vi "DMM.vi"(6 "Setting":T1={"Resolution (Digits)"=5.5, "Current Source (Amps)"=0.001, "Range"=2.0, "Measurement Type"=enum."DC Volts"} {"Resolution (Digits)" items=["3 1/2"=3.5, "4 1/2"=4.5, "5 1/2"=5.5, "6 1/2"=6.5, "7 1/2"=7.5]; "Current Source (Amps)" items=["1uA"=1e-06, "10uA"=1e-05, "100uA"=0.0001, "1mA"=0.001]}, 8 "error in":errorcluster, 9 "DMM Ref":string="NI_DMM_4072", 10 "DMM ClassName":string="NI DMM4072.lvclass", 11 "Base Path":path=path "C:/GitHub/OOP_OPC UA/Sequence/CodeModules/HAL/Concrete") -> (0 "error out":errorcluster={"status"=TRUE, "code"=-1073807346, "source"="VISA Open in APS-7000 Series.lvlib:Initialize.vi->Concrete.lvlib:APS7050.lvclass:Initialise.vi->Check objects.vi"}, 3 "Measurements":dbl)   [LabVIEW 2021]
uses:
  HAL/Harware Abstraction/MultiIO/DMM.lvclass
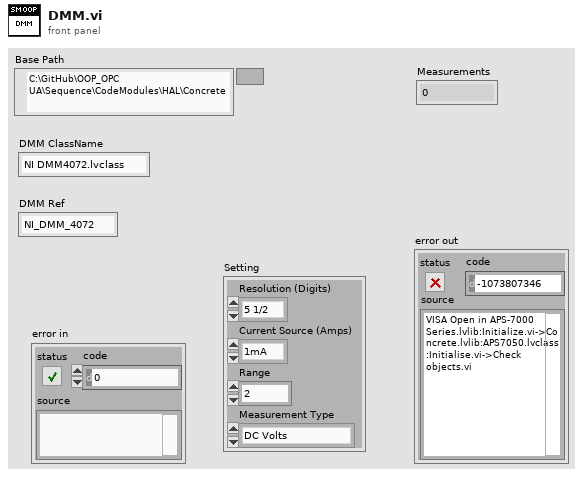
[diagram p1: front panel]
types:
  T1 = cluster{"Resolution (Digits)":dbl, "Current Source (Amps)":dbl, "Range":dbl, "Measurement Type":enum16{"DC Volts", "AC Volts", "DC Current", "AC Current", "2-wire Resistance", "4-wire Resistance", "Diode", "Frequency", "Period", "AC Volts DC Coupled", "Capacitance", "Inductance", "Temperature"}}
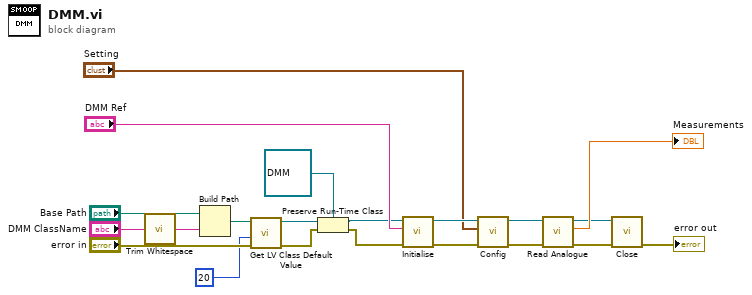
[diagram p0: block diagram]
diagram:
  n1 = call <vilib>:"Trim Whitespace.vi"("string"="DMM ClassName") -> ("trimmed string"=w18:string)  [unwired: 1 in]
  n2 = Build Path(base path="Base Path", name or relative path=w18) -> (appended path=w16:path)
  n3 = call <vilib>:"Get LV Class Default Value.vi"("error in (no error)"="error in", "options"=u32 20, "class path"=w16) -> ("error out"=w15:errorcluster, "object"=w19:refnum<class>)  [unwired: 7 in]
  n4 = Preserve Run-Time Class(object in=w19, error in=w15, 2:refnum<class "DMM.lvclass"> refnum ("HAL.lvlib:MultiFunction IO.lvclass")) -> (object out=w6:refnum<class "DMM.lvclass">, error out=w5:errorcluster)
  n5 = call-dynamic "Initialise.vi"("error in (no error)"=w5, "Instrument Ref"="DMM Ref", "Instrument in"=w6) -> ("error out"=w9:errorcluster, "Instrument out"=w11:refnum<class "DMM.lvclass">)  [unwired: 7 in]
  n6 = call-dynamic "Config.vi"("error in (no error)"=w9, "Setting"="Setting", "DMM in"=w11) -> ("error out"=w8:errorcluster, "DMM out"=w10:refnum<class "DMM.lvclass">)  [unwired: 7 in]
  n7 = call-dynamic "Read Analogue.vi"("error in (no error)"=w8, "DMM in"=w10) -> ("error out"=w13:errorcluster, "Measurement"=→"Measurements":dbl, "DMM out"=w12:refnum<class "DMM.lvclass">)  [unwired: 7 in]
  n8 = call-dynamic "Close.vi"("error in (no error)"=w13, "Instrument in"=w12) -> ("error out"=→"error out":errorcluster)  [unwired: 8 in, 1 out]
